vi "GetSoftwareVersion.vi"(8 "error in":errorcluster, 11 "VISA resource name":refnum<visa-resource-name>) -> (0 "error out":errorcluster, 2 "Software version":string, 3 "VISA resource name out":refnum<visa-resource-name>)   [LabVIEW 2023, in "Thermotron 8800.lvlib"]
doc: "VRSN\nCommand name: Send software version\nCommand type: System status\nDescription: Queries the 8800 for the version number of the display software.\nSyntax: VRSN?\nData type: String\nThe 8800 returns a string in the “Vx.yy dd/mm/yyyy” format to identify its software version.\nQuery example: VRSN?\n8800 response: V1.18 04/02/2005 (The software is version 1.18, released April 2, 2005.)"
uses:
  Thermotron 8800.lvlib
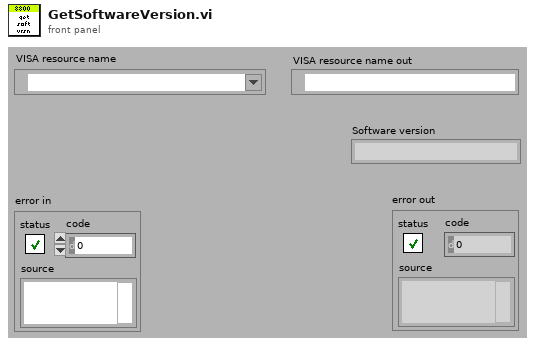
[diagram p1: front panel]
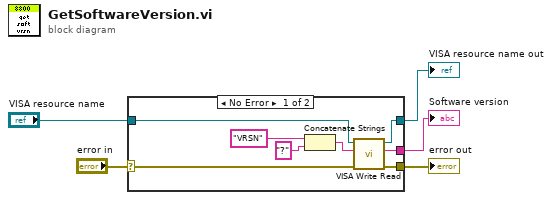
[diagram p0: block diagram]
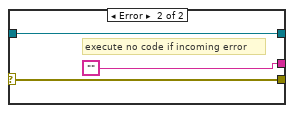
[diagram p2: hidden frame]
diagram:
  n1 = case shown="No Error" "error in" {
    selector: "error in" -> [w10 w15]
    tunnel: [w7 w15] -> w4
    tunnel: [w8 w16] -> w3
    tunnel: "VISA resource name" -> [w9 w16]
    tunnel: [w6 ""] -> w1
    frame No Error {
      n2 = Concatenate Strings("VRSN" ("8800 Command"), "?" ("8800 Command")) -> (w13:string)
      n3 = call "VISA Write Read.vi"("error in (no error)"=w10, "8800 Command"=w13, "VISA Refnum in"=w9) -> ("error out"=w7:errorcluster, "read buffer"=w6:string, "VISA Refnum out"=w8:refnum<visa-resource-name>)  [unwired: 6 in]
    }
    frame Error {
      # "execute no code if incoming error"
    }
  }
  "VISA resource name out" <- w3
  "error out" <- w4
  "Software version" <- w1
